vi "Slow Lift.vi"(8 "Encoder":dbl, 10 "Setpoint":dbl, 11 "Last Setpoint":dbl) -> (2 "Setpoint 2":dbl)   [LabVIEW 2014]
panel:
  in  "Speed (in/ms)":dbl=0.003 format="%#_13g"
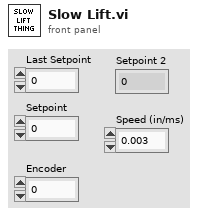
[diagram p1: front panel]
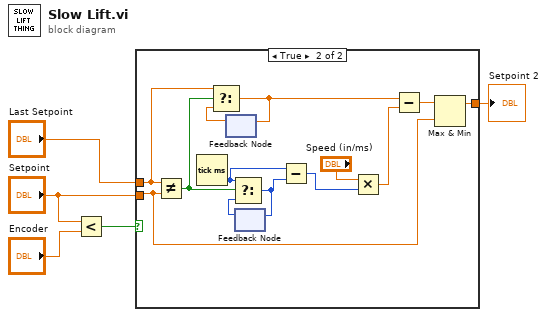
[diagram p0: block diagram]
diagram:
  n1 = Less?(x="Setpoint", y="Encoder") -> (x < y?=w4:bool)
  n2 = case shown="True" w4 {
    tunnel: "Setpoint" -> [w6 w12]
    tunnel: "Last Setpoint" -> [_ w18]
    tunnel: [w6 w10] -> w1
    frame False {
    }
    frame True {
      n3 = Not Equal?(x=w18, y=w12) -> (x != y?=w17:bool)
      n4 = Tick Count (ms)() -> (millisecond timer value=w9:u32)
      n5 = feedback #1() -> (w16:dbl)  [unwired: 1 in]
      n6 = Select(t=w18, s=w17, f=w16) -> (s? t:f=w11:dbl)
      n7 = feedback-in #1(w11) -> ()
      n8 = feedback #2() -> (w19:u32)  [unwired: 1 in]
      n9 = Select(t=w9, s=w17, f=w19) -> (s? t:f=w8:u32)
      n10 = feedback-in #2(w8) -> ()
      n11 = Subtract(x=w9, y=w8) -> (x-y=w7:u32)
      n12 = Multiply(x="Speed (in/ms)", y=w7) -> (x*y=w14:dbl)
      n13 = Subtract(x=w11, y=w14) -> (x-y=w13:dbl)
      n14 = Max & Min(x=w13, y=w12) -> (max(x,y)=w10:dbl)  [unwired: 1 out]
    }
  }
  "Setpoint 2" <- w1
